vi "Aktuell.vi"() -> ()   [LabVIEW 2012]
uses:
  <vilib>/NXT/Subs/MotorOutput.ctl
  <vilib>/NXT/NXT Controls/ConnectionType.ctl
  <vilib>/NXT/Block Support/NXT_InputPort.ctl
panel:
  out "?":bool
  out "?":bool
  out "?":bool
  out "?":bool
  out "?":bool
  out "Progress":u8(slide) scale=0.0..100.0
  out "Numeric 4":dbl
  out "Numeric 3":dbl
  out "Numeric 2":dbl
  out "Numeric":dbl
  in  "?":bool
  out "?":bool
  out "?":bool
  out "?":bool
  in  "MolekŸlnamen eingeben:":string
  out "Status:":string
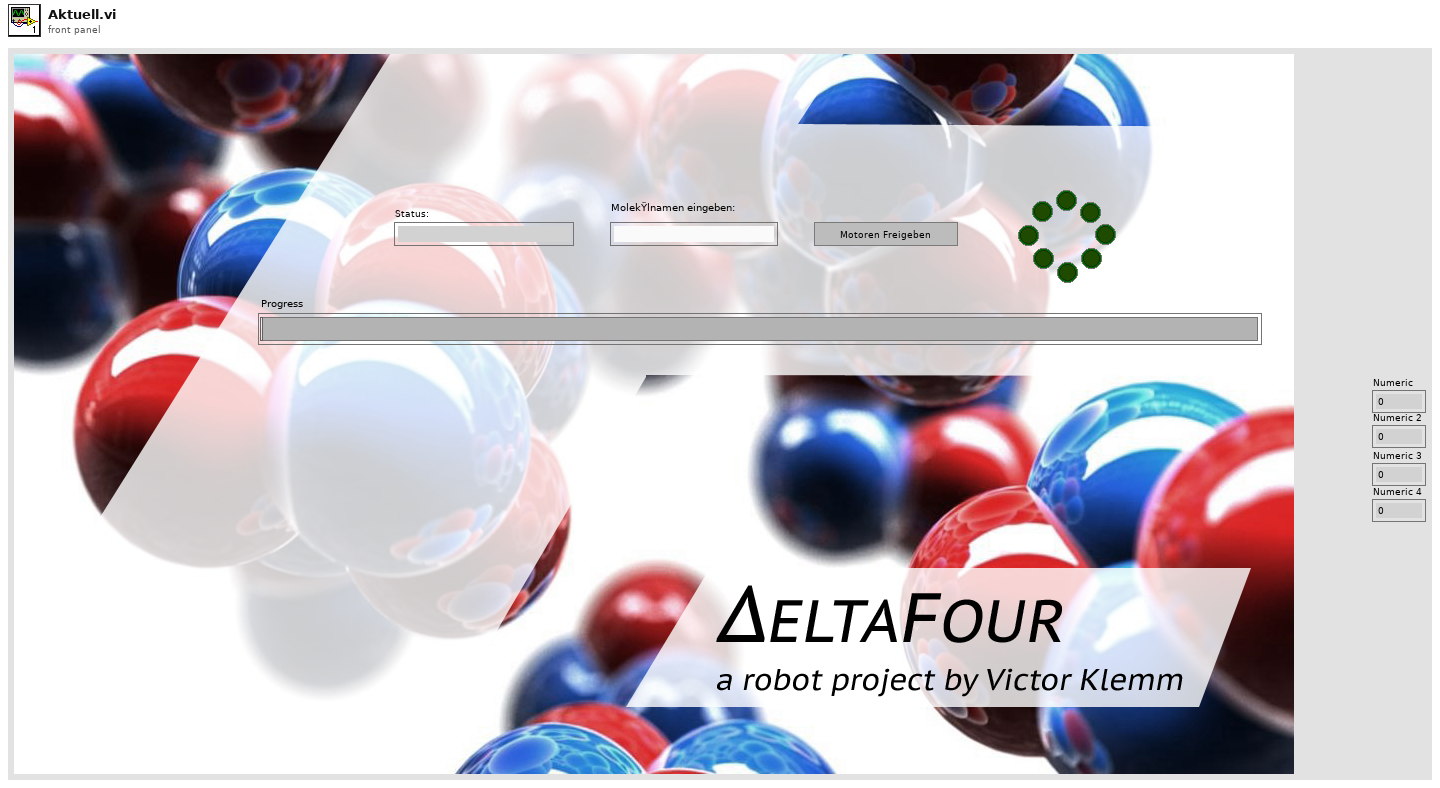
[diagram p1: front panel]
types:
  T1 = typedef "ConnectionType.ctl" = enum16{"Bluetooth", "USB", "WiFi"}
  T2 = typedef "LVHSConnector.ctl" = refnum<class "BrickReference.lvclass">
  T3 = typedef "MotorOutput.ctl" = u8
  T4 = typedef "NXT_InputPort.ctl" = u8
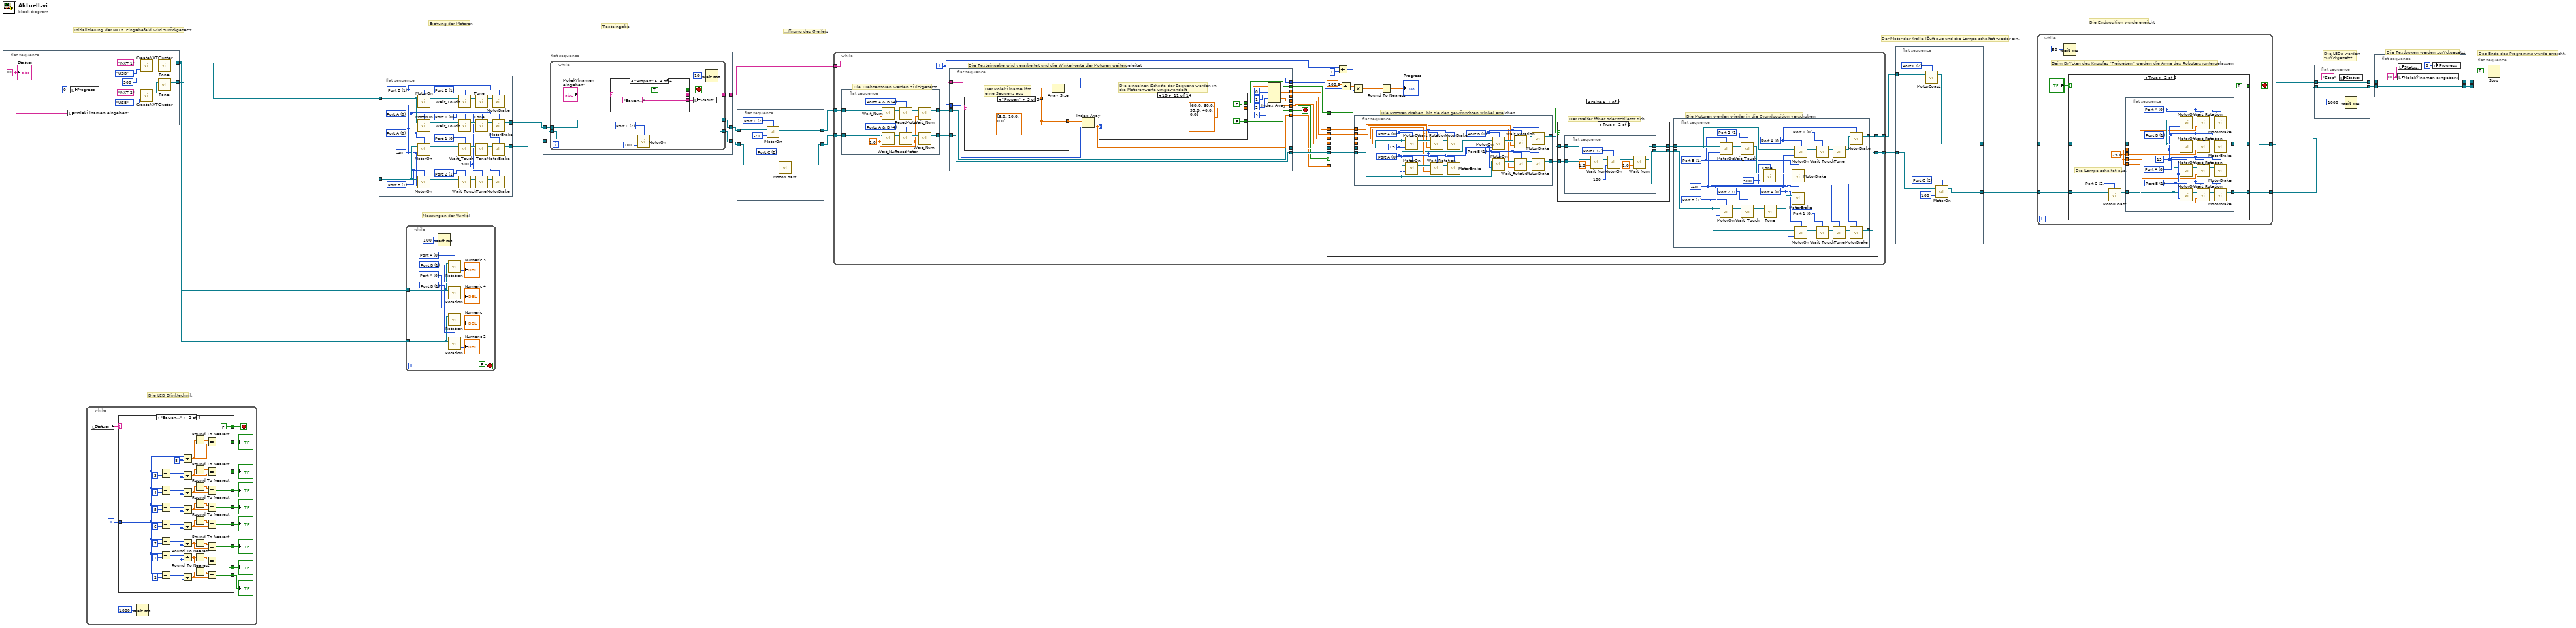
[diagram p0: block diagram]
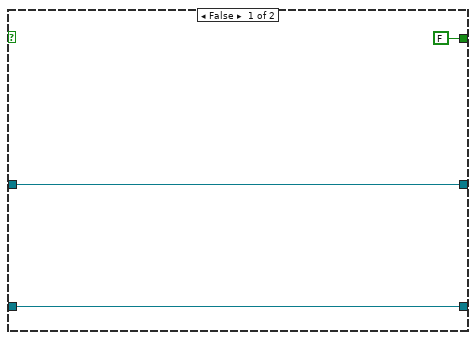
[diagram p2: hidden frame]
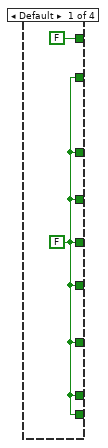
[diagram p3: hidden frame]
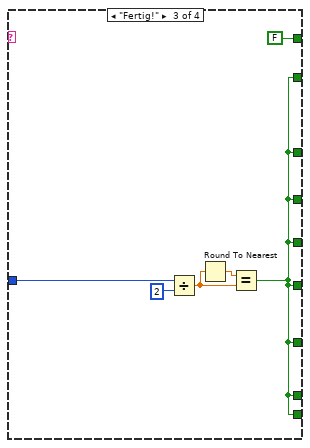
[diagram p4: hidden frame]
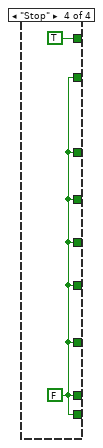
[diagram p5: hidden frame]
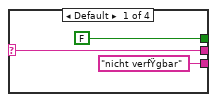
[diagram p6: hidden frame]
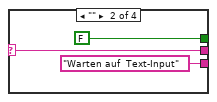
[diagram p7: hidden frame]
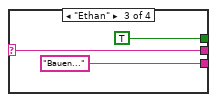
[diagram p8: hidden frame]
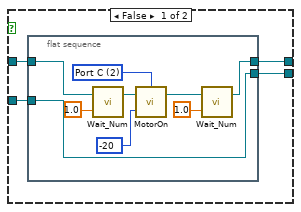
[diagram p9: hidden frame]
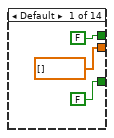
[diagram p11: hidden frame]
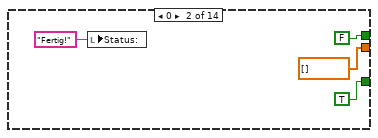
[diagram p12: hidden frame]
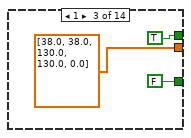
[diagram p13: hidden frame]
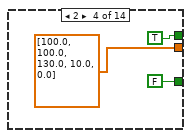
[diagram p14: hidden frame]
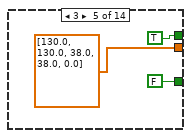
[diagram p15: hidden frame]
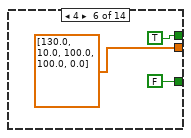
[diagram p16: hidden frame]
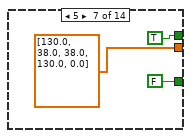
[diagram p17: hidden frame]
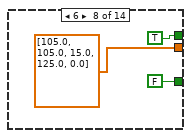
[diagram p18: hidden frame]
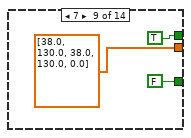
[diagram p19: hidden frame]
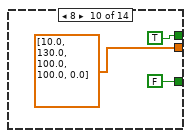
[diagram p20: hidden frame]
diagram:
  # "Der Motor der Kralle lŠuft aus und die Lampe schaltet wieder ein."
  # "Messungen der Winkel"
  # "Die LEDs werden\nzurŸckgesetzt"
  # "Die Textboxen werden zurŸckgesetzt"
  # "Das Ende des Programms wurde erreicht."
  # "Die Endposition wurde erreicht"
  # "…ffnung des Greifers"
  # "Texteingabe"
  # "Eichung der Motoren"
  # "Initialisierung der NXTs. Eingabefeld wird zurŸckgesetzt."
  # "Die LED Blinktechnik"
  n1 = flat-sequence {
    tunnel: [w27] -> w4
    tunnel: [w25] -> w5
    frame #0 {
      w24 = "" ("Status:")
      n2 = local write "MolekŸlnamen eingeben:"(w24) -> ()
      n3 = local write "Progress"(u8 0 ("Progress")) -> ()
      n4 = call <vilib>:"CreateNXTCluster.vi"("Connection Type"=ConnectionType."USB", "NXT name"="NXT 1") -> ("NXT"=w28:T2)  [unwired: 2 in]
      n5 = call <vilib>:"CreateNXTCluster.vi"("Connection Type"=ConnectionType."USB", "NXT name"="NXT 2") -> ("NXT"=w26:T2)  [unwired: 2 in]
      n6 = call <vilib>:"Tone.vi"("NXT"=w28) -> ("NXT"=w27:T2)  [unwired: 3 in]
      n7 = call <vilib>:"Tone.vi"("NXT"=w26, "Tone (440 Hz)"=u16 500) -> ("NXT"=w25:T2)  [unwired: 2 in]
      "Status:" <- w24
    }
  }
  n8 = while {
    i -> [w42]
    stop <- w40 stop-if-true
    n9 = local read "Status:"() -> (w39:string)
    n10 = case shown="\"Bauen...\"" w39 {
      tunnel: w42 -> [_ w46 w88 _]
      tunnel: [FALSE FALSE FALSE TRUE] -> w40
      tunnel: [w43 w74 w86 w92] -> w38
      tunnel: [w43 w73 w86 w92] -> w37
      tunnel: [w43 w72 w86 w92] -> w36
      tunnel: [w43 w67 w86 w92] -> w35
      tunnel: [w43 w63 w86 w92] -> w34
      tunnel: [w43 w57 w86 w92] -> w33
      tunnel: [w43 w52 w86 w92] -> w32
      tunnel: [w43 w47 w86 w92] -> w31
      frame Default {
        w43 = FALSE ("stop? (T)")
      }
      frame "Bauen..." {
        w45 = 8 ("y")
        n11 = Subtract(x=w46, y=3) -> (x-y=w69:i32)
        n12 = Subtract(x=w46, y=4) -> (x-y=w65:i32)
        n13 = Subtract(x=w46, y=5) -> (x-y=w60:i32)
        n14 = Subtract(x=w46, y=6) -> (x-y=w55:i32)
        n15 = Subtract(x=w46, y=7) -> (x-y=w50:i32)
        n16 = Subtract(x=w46, y=1) -> (x-y=w81:i32)
        n17 = Subtract(x=w46, y=2) -> (x-y=w77:i32)
        n18 = Divide(x=w46, y=w45) -> (x/y=w84:dbl)
        n19 = Divide(x=w69, y=w45) -> (x/y=w70:dbl)
        n20 = Divide(x=w65, y=w45) -> (x/y=w66:dbl)
        n21 = Divide(x=w60, y=w45) -> (x/y=w61:dbl)
        n22 = Divide(x=w55, y=w45) -> (x/y=w56:dbl)
        n23 = Divide(x=w50, y=w45) -> (x/y=w51:dbl)
        n24 = Divide(x=w81, y=w45) -> (x/y=w82:dbl)
        n25 = Divide(x=w77, y=w45) -> (x/y=w78:dbl)
        n26 = Round To Nearest(number=w84) -> (nearest integer value=w85:dbl)
        n27 = Round To Nearest(number=w70) -> (nearest integer value=w71:dbl)
        n28 = Round To Nearest(number=w66) -> (nearest integer value=w62:dbl)
        n29 = Round To Nearest(number=w61) -> (nearest integer value=w58:dbl)
        n30 = Round To Nearest(number=w56) -> (nearest integer value=w53:dbl)
        n31 = Round To Nearest(number=w51) -> (nearest integer value=w48:dbl)
        n32 = Round To Nearest(number=w82) -> (nearest integer value=w83:dbl)
        n33 = Round To Nearest(number=w78) -> (nearest integer value=w79:dbl)
        n34 = Equal?(x=w85, y=w84) -> (x = y?=w74:bool)
        n35 = Equal?(x=w71, y=w70) -> (x = y?=w67:bool)
        n36 = Equal?(x=w62, y=w66) -> (x = y?=w63:bool)
        n37 = Equal?(x=w58, y=w61) -> (x = y?=w57:bool)
        n38 = Equal?(x=w53, y=w56) -> (x = y?=w52:bool)
        n39 = Equal?(x=w48, y=w51) -> (x = y?=w47:bool)
        n40 = Equal?(x=w83, y=w82) -> (x = y?=w72:bool)
        n41 = Equal?(x=w79, y=w78) -> (x = y?=w73:bool)
      }
      frame "Fertig!" {
        n42 = Divide(x=w88, y=2) -> (x/y=w90:dbl)
        n43 = Round To Nearest(number=w90) -> (nearest integer value=w87:dbl)
        n44 = Equal?(x=w87, y=w90) -> (x = y?=w86:bool)
      }
      frame "Stop" {
        w92 = FALSE ("stop? (T)")
      }
    }
    "?" <- w38
    "?" <- w37
    "?" <- w36
    "?" <- w32
    "?" <- w31
    "?" <- w35
    "?" <- w34
    "?" <- w33
    n45 = Wait (ms)(milliseconds to wait=u32 1000) -> ()  [unwired: 1 out]
  }
  n46 = flat-sequence {
    tunnel: w5 -> [w115]
    tunnel: w4 -> [w114]
    tunnel: [w101] -> w9
    tunnel: [w100] -> w6
    frame #0 {
      w94 = u16 500 ("Tone (440 Hz)")
      w97 = T3 1 items=["Port A"=0, "Port B"=1, "Port C"=2, "Ports A & B"=4, "Ports A & C"=5, "Ports B & C"=6, "All Ports"=3] ("Output Port (All Ports)")
      w110 = T4 1 items=["Port 1", "Port 2", "Port 3", "Port 4"] ("Port (Port 1)")
      w109 = T4 0 items=["Port 1", "Port 2", "Port 3", "Port 4"] ("Port (Port 1)")
      w95 = T3 1 items=["Port A"=0, "Port B"=1, "Port C"=2, "Ports A & B"=4, "Ports A & C"=5, "Ports B & C"=6, "All Ports"=3] ("Output Port (All Ports)")
      w96 = T3 0 items=["Port A"=0, "Port B"=1, "Port C"=2, "Ports A & B"=4, "Ports A & C"=5, "Ports B & C"=6, "All Ports"=3] ("Output Port (All Ports)")
      w98 = T4 1 items=["Port 1", "Port 2", "Port 3", "Port 4"] ("Port (Port 1)")
      w111 = T4 0 items=["Port 1", "Port 2", "Port 3", "Port 4"] ("Port (Port 1)")
      w102 = -40 ("Power (75)")
      w99 = T3 0 items=["Port A"=0, "Port B"=1, "Port C"=2, "Ports A & B"=4, "Ports A & C"=5, "Ports B & C"=6, "All Ports"=3] ("Output Port (All Ports)")
      n47 = call <vilib>:"MotorOn.vi"("Power (75)"=w102, "NXT"=w114, "Output Port (All Ports)"=w95) -> ("NXT"=w116:T2)  [unwired: 1 in]
      n48 = call <vilib>:"MotorOn.vi"("Power (75)"=w102, "NXT"=w114, "Output Port (All Ports)"=w96) -> ("NXT"=w117:T2)  [unwired: 1 in]
      n49 = call <vilib>:"MotorOn.vi"("Power (75)"=w102, "NXT"=w115, "Output Port (All Ports)"=w99) -> ("NXT"=w119:T2)  [unwired: 1 in]
      n50 = call <vilib>:"MotorOn.vi"("Power (75)"=w102, "NXT"=w115, "Output Port (All Ports)"=w97) -> ("NXT"=w118:T2)  [unwired: 1 in]
      n51 = call <vilib>:"Wait_Touch.vi"("NXT"=w116, "Port (Port 1)"=w110) -> ("NXT"=w106:T2)  [unwired: 2 in]
      n52 = call <vilib>:"Wait_Touch.vi"("NXT"=w117, "Port (Port 1)"=w109) -> ("NXT"=w104:T2)  [unwired: 2 in]
      n53 = call <vilib>:"Wait_Touch.vi"("NXT"=w119, "Port (Port 1)"=w111) -> ("NXT"=w113:T2)  [unwired: 2 in]
      n54 = call <vilib>:"Wait_Touch.vi"("NXT"=w118, "Port (Port 1)"=w98) -> ("NXT"=w108:T2)  [unwired: 2 in]
      n55 = call <vilib>:"Tone.vi"("NXT"=w106) -> ("NXT"=w105:T2)  [unwired: 3 in]
      n56 = call <vilib>:"Tone.vi"("NXT"=w104, "Tone (440 Hz)"=w94) -> ("NXT"=w103:T2)  [unwired: 2 in]
      n57 = call <vilib>:"Tone.vi"("NXT"=w113) -> ("NXT"=w112:T2)  [unwired: 3 in]
      n58 = call <vilib>:"Tone.vi"("NXT"=w108, "Tone (440 Hz)"=w94) -> ("NXT"=w107:T2)  [unwired: 2 in]
      n59 = call <vilib>:"MotorBrake.vi"("NXT"=w105, "Port (All Ports)"=w95) -> ()  [unwired: 2 in, 1 out]
      n60 = call <vilib>:"MotorBrake.vi"("NXT"=w103, "Port (All Ports)"=w96) -> ("NXT"=w100:T2)  [unwired: 2 in]
      n61 = call <vilib>:"MotorBrake.vi"("NXT"=w112, "Port (All Ports)"=w99) -> ("NXT"=w101:T2)  [unwired: 2 in]
      n62 = call <vilib>:"MotorBrake.vi"("NXT"=w107, "Port (All Ports)"=w97) -> ()  [unwired: 2 in, 1 out]
    }
  }
  n63 = while {
    tunnel: w5 -> [w127]
    tunnel: w4 -> [w126]
    stop <- FALSE stop-if-true
    w129 = T3 1 items=["Port A"=0, "Port B"=1, "Port C"=2, "Ports A & B"=4, "Ports A & C"=5, "Ports B & C"=6, "All Ports"=3] ("Output Port (All Ports)")
    w128 = T3 0 items=["Port A"=0, "Port B"=1, "Port C"=2, "Ports A & B"=4, "Ports A & C"=5, "Ports B & C"=6, "All Ports"=3] ("Output Port (All Ports)")
    w131 = T3 1 items=["Port A"=0, "Port B"=1, "Port C"=2, "Ports A & B"=4, "Ports A & C"=5, "Ports B & C"=6, "All Ports"=3] ("Output Port (All Ports)")
    w130 = T3 0 items=["Port A"=0, "Port B"=1, "Port C"=2, "Ports A & B"=4, "Ports A & C"=5, "Ports B & C"=6, "All Ports"=3] ("Output Port (All Ports)")
    n64 = Wait (ms)(milliseconds to wait=u32 100) -> ()  [unwired: 1 out]
    n65 = call <vilib>:"Rotation.vi"("NXT"=w127, "Port (Port A)"=w130) -> ("Angle of Rotation"=→"Numeric 3":i32)  [unwired: 1 in, 1 out]
    n66 = call <vilib>:"Rotation.vi"("NXT"=w127, "Port (Port A)"=w131) -> ("Angle of Rotation"=→"Numeric 4":i32)  [unwired: 1 in, 1 out]
    n67 = call <vilib>:"Rotation.vi"("NXT"=w126, "Port (Port A)"=w128) -> ("Angle of Rotation"=→"Numeric":i32)  [unwired: 1 in, 1 out]
    n68 = call <vilib>:"Rotation.vi"("NXT"=w126, "Port (Port A)"=w129) -> ("Angle of Rotation"=→"Numeric 2":i32)  [unwired: 1 in, 1 out]
  }
  n69 = flat-sequence {
    tunnel: w6 -> [w134]
    tunnel: [w136] -> w19
    tunnel: [w135] -> w18
    tunnel: [w132] -> w17
    tunnel: w9 -> [w133]
    frame #0 {
      n70 = while {
        tunnel: [w144] -> w136
        tunnel: [w141] -> w135
        tunnel: w134 -> [w141]
        tunnel: w133 -> [w138]
        tunnel: [w137] -> w132
        stop <- w142 stop-if-true
        w140 = T3 2 items=["Port A"=0, "Port B"=1, "Port C"=2, "Ports A & B"=4, "Ports A & C"=5, "Ports B & C"=6, "All Ports"=3] ("Output Port (All Ports)")
        n71 = case shown="\"Propan\"" "MolekŸlnamen eingeben:" {
          selector: "MolekŸlnamen eingeben:" -> [w148 w152 w155 w158]
          tunnel: [FALSE FALSE TRUE TRUE] -> w142
          tunnel: [w148 w152 w155 w158] -> w144
          tunnel: ["nicht verfŸgbar" ("Status") "Warten auf  Text-Input" ("Status") "Bauen..." ("Status") "Bauen..." ("Status")] -> w143
          frame Default {
          }
          frame "" {
          }
          frame "Ethan" {
          }
          frame "Propan" {
          }
        }
        n72 = call <vilib>:"MotorOn.vi"("Power (75)"=100, "NXT"=w138, "Output Port (All Ports)"=w140) -> ("NXT"=w137:T2)  [unwired: 1 in]
        n73 = local write "Status:"(w143) -> ()
        n74 = Wait (ms)(milliseconds to wait=u32 10) -> ()  [unwired: 1 out]
      }
    }
  }
  n75 = flat-sequence {
    tunnel: w18 -> [w162]
    tunnel: [w163] -> w8
    tunnel: [w160] -> w7
    tunnel: w17 -> [w161]
    frame #0 {
      w159 = T3 2 items=["Port A"=0, "Port B"=1, "Port C"=2, "Ports A & B"=4, "Ports A & C"=5, "Ports B & C"=6, "All Ports"=3] ("Port (All Ports)")
      w164 = T3 2 items=["Port A"=0, "Port B"=1, "Port C"=2, "Ports A & B"=4, "Ports A & C"=5, "Ports B & C"=6, "All Ports"=3] ("Output Port (All Ports)")
      n76 = call <vilib>:"MotorOn.vi"("Power (75)"=-20, "NXT"=w162, "Output Port (All Ports)"=w164) -> ("NXT"=w163:T2)  [unwired: 1 in]
      n77 = call <vilib>:"MotorCoast.vi"("NXT"=w161, "Port (All Ports)"=w159) -> ("NXT"=w160:T2)  [unwired: 2 in]
    }
  }
  n78 = while {
    tunnel: w8 -> [w183]
    tunnel: w7 -> [w182]
    tunnel: w19 -> [w179]
    tunnel: [w175] -> w16
    tunnel: [w176] -> w3
    i -> [w168]
    stop <- w177 stop-if-true
    # "Die Texteingabe wird verarbeitet und die Winkelwerte der Motoren weitergeleitet"
    # "Die Drehsensoren werden zŸrickgesetzt"
    n79 = flat-sequence {
      tunnel: w183 -> [w350]
      tunnel: [w345] -> w181
      tunnel: [w344] -> w180
      tunnel: w182 -> [w343]
      frame #0 {
        w346 = sgl 1.0 ("Time (1 sec)")
        w352 = T3 4 items=["Port A"=0, "Port B"=1, "Port C"=2, "Ports A & B"=4, "Ports A & C"=5, "Ports B & C"=6, "All Ports"=3] ("Port (All Ports)")
        w353 = T3 4 items=["Port A"=0, "Port B"=1, "Port C"=2, "Ports A & B"=4, "Ports A & C"=5, "Ports B & C"=6, "All Ports"=3] ("Port (All Ports)")
        n80 = call <vilib>:"Wait_Num.vi"("Time (1 sec)"=w346, "NXT"=w350) -> ("NXT"=w349:T2)  [unwired: 2 in]
        n81 = call <vilib>:"Wait_Num.vi"("Time (1 sec)"=w346, "NXT"=w343) -> ("NXT"=w351:T2)  [unwired: 2 in]
        n82 = call <vilib>:"ResetMotor.vi"("NXT"=w349, "Port (All Ports)"=w353) -> ("NXT"=w348:T2)  [unwired: 2 in]
        n83 = call <vilib>:"ResetMotor.vi"("NXT"=w351, "Port (All Ports)"=w352) -> ("NXT"=w347:T2)  [unwired: 2 in]
        n84 = call <vilib>:"Wait_Num.vi"("Time (1 sec)"=w346, "NXT"=w348) -> ("NXT"=w345:T2)  [unwired: 2 in]
        n85 = call <vilib>:"Wait_Num.vi"("Time (1 sec)"=w346, "NXT"=w347) -> ("NXT"=w344:T2)  [unwired: 2 in]
      }
    }
    n86 = flat-sequence {
      tunnel: [w292] -> w189
      tunnel: [w291] -> w188
      tunnel: [w290] -> w187
      tunnel: [w289] -> w186
      tunnel: [w284] -> w185
      tunnel: w181 -> [w284]
      tunnel: w180 -> [w288]
      tunnel: [w288] -> w184
      tunnel: w179 -> [w287]
      tunnel: w168 -> [w281]
      tunnel: [w285] -> w177
      tunnel: [w282] -> w178
      tunnel: [w280] -> w174
      tunnel: [w278] -> w169
      frame #0 {
        # "Die einzelnen Schritte der Sequenz werden in\ndie Motorenwerte umgewandelt"
        # "Der MolekŸlname lšst eine Sequenz aus"
        n87 = case shown="\"Propan\"" w287 {
          tunnel: [w340 w341 w342] -> w286
          tunnel: [w340 w341 w342] -> w279
          frame Default {
            w340 = dbl[] [0.0] ("array")
          }
          frame "Ethan" {
            w341 = dbl[] [8.0, 10.0, 2.0, 11.0, 0.0] ("array")
          }
          frame "Propan" {
            w342 = dbl[] [6.0, 10.0, 0.0] ("array")
          }
        }
        n88 = Array Size(array=w279) -> (size(s)=w278:i32)
        n89 = Index Array(array=w286, index=w281) -> (element=w280:dbl)
        n90 = case shown="10" w280 {
          tunnel: [FALSE TRUE FALSE FALSE FALSE FALSE FALSE FALSE FALSE FALSE FALSE FALSE FALSE FALSE] -> w285
          tunnel: [dbl[] [] ("array") dbl[] [] ("array") dbl[] [38.0, 38.0, 130.0, 130.0, 0.0] ("array") dbl[] [100.0, 100.0, 130.0, 10.0, 0.0] ("array") dbl[] [130.0, 130.0, 38.0, 38.0, 0.0] ("array") dbl[] [130.0, 10.0, 100.0, 100.0, 0.0] ("array") dbl[] [130.0, 38.0, 38.0, 130.0, 0.0] ("array") dbl[] [105.0, 105.0, 15.0, 125.0, 0.0] ("array") dbl[] [38.0, 130.0, 38.0, 130.0, 0.0] ("array") dbl[] [10.0, 130.0, 100.0, 100.0, 0.0] ("array") dbl[] [60.0, 60.0, 35.0, 40.0, 0.0] ("array") dbl[] [0.0, 0.0, 0.0, 0.0, 0.0] ("array") dbl[] [0.0, 0.0, 0.0, 0.0, 0.0] ("array") dbl[] [0.0, 0.0, 0.0, 0.0, 0.0] ("array")] -> w283
          tunnel: [FALSE FALSE TRUE TRUE TRUE TRUE TRUE TRUE TRUE TRUE FALSE FALSE FALSE FALSE] -> w282
          frame Default {
          }
          frame 0 {
            n91 = local write "Status:"("Fertig!" ("Status:")) -> ()
          }
          frame 1 {
          }
          frame 2 {
          }
          frame 3 {
          }
          frame 4 {
          }
          frame 5 {
          }
          frame 6 {
          }
          frame 7 {
          }
          frame 8 {
          }
          frame 10 {
          }
          frame 11 {
          }
          frame 12 {
          }
          frame 13 {
          }
        }
        n92 = Index Array(array=w283, index #1=0 ("index"), index #2=1 ("index"), index #3=2 ("index"), index #4=3 ("index")) -> (element #1=w291:dbl, element #2=w290:dbl, element #3=w289:dbl, element #4=w292:dbl)
      }
    }
    n93 = case shown="False" w177 {
      tunnel: w189 -> [w196 _]
      tunnel: w188 -> [w199 _]
      tunnel: w187 -> [w198 _]
      tunnel: w186 -> [w197 _]
      tunnel: w185 -> [w195 w277]
      tunnel: w184 -> [w194 w276]
      tunnel: [w193 w277] -> w175
      tunnel: [w192 w276] -> w176
      tunnel: w178 -> [w200 _]
      tunnel: w174 -> [_ _]
      frame False {
        # "Die Motoren drehen, bis sie den gewŸnschten Winkel erreichen"
        # "Der Greifer šffnet oder schliesst sich"
        # "Die Motoren werden wieder in die Grundposition verschoben"
        n94 = flat-sequence {
          tunnel: w194 -> [w249]
          tunnel: w195 -> [w229]
          tunnel: [w236] -> w201
          tunnel: [w235] -> w202
          tunnel: w199 -> [w233]
          tunnel: w198 -> [w232]
          tunnel: w197 -> [w231]
          tunnel: w196 -> [w230]
          frame #0 {
            w234 = 15 ("Power (75)")
            w240 = T3 1 items=["Port A"=0, "Port B"=1, "Port C"=2, "Ports A & B"=4, "Ports A & C"=5, "Ports B & C"=6, "All Ports"=3] ("Output Port (All Ports)")
            w239 = T3 0 items=["Port A"=0, "Port B"=1, "Port C"=2, "Ports A & B"=4, "Ports A & C"=5, "Ports B & C"=6, "All Ports"=3] ("Output Port (All Ports)")
            w237 = T3 1 items=["Port A"=0, "Port B"=1, "Port C"=2, "Ports A & B"=4, "Ports A & C"=5, "Ports B & C"=6, "All Ports"=3] ("Output Port (All Ports)")
            w241 = T3 0 items=["Port A"=0, "Port B"=1, "Port C"=2, "Ports A & B"=4, "Ports A & C"=5, "Ports B & C"=6, "All Ports"=3] ("Output Port (All Ports)")
            n95 = call <vilib>:"MotorOn.vi"("Power (75)"=w234, "NXT"=w229, "Output Port (All Ports)"=w239) -> ("NXT"=w246:T2)  [unwired: 1 in]
            n96 = call <vilib>:"MotorOn.vi"("Power (75)"=w234, "NXT"=w249, "Output Port (All Ports)"=w241) -> ("NXT"=w248:T2)  [unwired: 1 in]
            n97 = call <vilib>:"Wait_Rotation.vi"("Position Change (180)"=w233, "NXT"=w246, "Port (Port A)"=w239) -> ("NXT"=w244:T2)  [unwired: 1 in]
            n98 = call <vilib>:"Wait_Rotation.vi"("Position Change (180)"=w231, "NXT"=w248, "Port (Port A)"=w241) -> ("NXT"=w242:T2)  [unwired: 1 in]
            n99 = call <vilib>:"MotorBrake.vi"("NXT"=w244, "Port (All Ports)"=w239) -> ()  [unwired: 2 in, 1 out]
            n100 = call <vilib>:"MotorBrake.vi"("NXT"=w242, "Port (All Ports)"=w241) -> ()  [unwired: 2 in, 1 out]
            n101 = call <vilib>:"MotorOn.vi"("Power (75)"=w234, "NXT"=w229, "Output Port (All Ports)"=w240) -> ("NXT"=w247:T2)  [unwired: 1 in]
            n102 = call <vilib>:"MotorOn.vi"("Power (75)"=w234, "NXT"=w249, "Output Port (All Ports)"=w237) -> ("NXT"=w245:T2)  [unwired: 1 in]
            n103 = call <vilib>:"Wait_Rotation.vi"("Position Change (180)"=w232, "NXT"=w247, "Port (Port A)"=w240) -> ("NXT"=w243:T2)  [unwired: 1 in]
            n104 = call <vilib>:"Wait_Rotation.vi"("Position Change (180)"=w230, "NXT"=w245, "Port (Port A)"=w237) -> ("NXT"=w238:T2)  [unwired: 1 in]
            n105 = call <vilib>:"MotorBrake.vi"("NXT"=w243, "Port (All Ports)"=w240) -> ("NXT"=w235:T2)  [unwired: 2 in]
            n106 = call <vilib>:"MotorBrake.vi"("NXT"=w238, "Port (All Ports)"=w237) -> ("NXT"=w236:T2)  [unwired: 2 in]
          }
        }
        n107 = case shown="True" w200 {
          tunnel: w202 -> [w206 w219]
          tunnel: w201 -> [w205 w218]
          tunnel: [w204 w217] -> w191
          tunnel: [w203 w216] -> w190
          frame False {
            n108 = flat-sequence {
              tunnel: [w207] -> w204
              tunnel: [w210] -> w203
              tunnel: w206 -> [w212]
              tunnel: w205 -> [w210]
              frame #0 {
                w214 = T3 2 items=["Port A"=0, "Port B"=1, "Port C"=2, "Ports A & B"=4, "Ports A & C"=5, "Ports B & C"=6, "All Ports"=3] ("Output Port (All Ports)")
                n109 = call <vilib>:"Wait_Num.vi"("Time (1 sec)"=sgl 1.0, "NXT"=w212) -> ("NXT"=w211:T2)  [unwired: 2 in]
                n110 = call <vilib>:"MotorOn.vi"("Power (75)"=-20, "NXT"=w211, "Output Port (All Ports)"=w214) -> ("NXT"=w208:T2)  [unwired: 1 in]
                n111 = call <vilib>:"Wait_Num.vi"("Time (1 sec)"=sgl 1.0, "NXT"=w208) -> ("NXT"=w207:T2)  [unwired: 2 in]
              }
            }
          }
          frame True {
            n112 = flat-sequence {
              tunnel: w218 -> [w222]
              tunnel: [w221] -> w217
              tunnel: w219 -> [w225]
              tunnel: [w222] -> w216
              frame #0 {
                w226 = T3 2 items=["Port A"=0, "Port B"=1, "Port C"=2, "Ports A & B"=4, "Ports A & C"=5, "Ports B & C"=6, "All Ports"=3] ("Output Port (All Ports)")
                n113 = call <vilib>:"Wait_Num.vi"("Time (1 sec)"=sgl 1.0, "NXT"=w225) -> ("NXT"=w224:T2)  [unwired: 2 in]
                n114 = call <vilib>:"MotorOn.vi"("Power (75)"=100, "NXT"=w224, "Output Port (All Ports)"=w226) -> ("NXT"=w220:T2)  [unwired: 1 in]
                n115 = call <vilib>:"Wait_Num.vi"("Time (1 sec)"=sgl 1.0, "NXT"=w220) -> ("NXT"=w221:T2)  [unwired: 2 in]
              }
            }
          }
        }
        n116 = flat-sequence {
          tunnel: w191 -> [w271]
          tunnel: w190 -> [w270]
          tunnel: [w257] -> w193
          tunnel: [w256] -> w192
          frame #0 {
            w250 = u16 500 ("Tone (440 Hz)")
            w253 = T3 1 items=["Port A"=0, "Port B"=1, "Port C"=2, "Ports A & B"=4, "Ports A & C"=5, "Ports B & C"=6, "All Ports"=3] ("Output Port (All Ports)")
            w266 = T4 1 items=["Port 1", "Port 2", "Port 3", "Port 4"] ("Port (Port 1)")
            w265 = T4 0 items=["Port 1", "Port 2", "Port 3", "Port 4"] ("Port (Port 1)")
            w251 = T3 1 items=["Port A"=0, "Port B"=1, "Port C"=2, "Ports A & B"=4, "Ports A & C"=5, "Ports B & C"=6, "All Ports"=3] ("Output Port (All Ports)")
            w252 = T3 0 items=["Port A"=0, "Port B"=1, "Port C"=2, "Ports A & B"=4, "Ports A & C"=5, "Ports B & C"=6, "All Ports"=3] ("Output Port (All Ports)")
            w254 = T4 1 items=["Port 1", "Port 2", "Port 3", "Port 4"] ("Port (Port 1)")
            w267 = T4 0 items=["Port 1", "Port 2", "Port 3", "Port 4"] ("Port (Port 1)")
            w258 = -40 ("Power (75)")
            w255 = T3 0 items=["Port A"=0, "Port B"=1, "Port C"=2, "Ports A & B"=4, "Ports A & C"=5, "Ports B & C"=6, "All Ports"=3] ("Output Port (All Ports)")
            n117 = call <vilib>:"MotorOn.vi"("Power (75)"=w258, "NXT"=w271, "Output Port (All Ports)"=w253) -> ("NXT"=w274:T2)  [unwired: 1 in]
            n118 = call <vilib>:"MotorOn.vi"("Power (75)"=w258, "NXT"=w270, "Output Port (All Ports)"=w251) -> ("NXT"=w272:T2)  [unwired: 1 in]
            n119 = call <vilib>:"Wait_Touch.vi"("NXT"=w274, "Port (Port 1)"=w254) -> ("NXT"=w264:T2)  [unwired: 2 in]
            n120 = call <vilib>:"Wait_Touch.vi"("NXT"=w272, "Port (Port 1)"=w266) -> ("NXT"=w262:T2)  [unwired: 2 in]
            n121 = call <vilib>:"Tone.vi"("NXT"=w264, "Tone (440 Hz)"=w250) -> ("NXT"=w263:T2)  [unwired: 2 in]
            n122 = call <vilib>:"Tone.vi"("NXT"=w262) -> ("NXT"=w261:T2)  [unwired: 3 in]
            n123 = call <vilib>:"MotorBrake.vi"("NXT"=w263, "Port (All Ports)"=w253) -> ()  [unwired: 2 in, 1 out]
            n124 = call <vilib>:"MotorBrake.vi"("NXT"=w261, "Port (All Ports)"=w251) -> ()  [unwired: 2 in, 1 out]
            n125 = call <vilib>:"MotorOn.vi"("Power (75)"=w258, "NXT"=w271, "Output Port (All Ports)"=w255) -> ("NXT"=w275:T2)  [unwired: 1 in]
            n126 = call <vilib>:"MotorOn.vi"("Power (75)"=w258, "NXT"=w270, "Output Port (All Ports)"=w252) -> ("NXT"=w273:T2)  [unwired: 1 in]
            n127 = call <vilib>:"Wait_Touch.vi"("NXT"=w275, "Port (Port 1)"=w267) -> ("NXT"=w269:T2)  [unwired: 2 in]
            n128 = call <vilib>:"Wait_Touch.vi"("NXT"=w273, "Port (Port 1)"=w265) -> ("NXT"=w260:T2)  [unwired: 2 in]
            n129 = call <vilib>:"Tone.vi"("NXT"=w269) -> ("NXT"=w268:T2)  [unwired: 3 in]
            n130 = call <vilib>:"Tone.vi"("NXT"=w260, "Tone (440 Hz)"=w250) -> ("NXT"=w259:T2)  [unwired: 2 in]
            n131 = call <vilib>:"MotorBrake.vi"("NXT"=w268, "Port (All Ports)"=w255) -> ("NXT"=w257:T2)  [unwired: 2 in]
            n132 = call <vilib>:"MotorBrake.vi"("NXT"=w259, "Port (All Ports)"=w252) -> ("NXT"=w256:T2)  [unwired: 2 in]
          }
        }
      }
      frame True {
      }
    }
    n133 = Add(x=w168, y=1) -> (x+y=w166:i32)
    n134 = Divide(x=100.0 ("y"), y=w169) -> (x/y=w172:dbl)
    n135 = Multiply(x=w172, y=w166) -> (x*y=w171:dbl)
    n136 = Round To Nearest(number=w171) -> (nearest integer value=→"Progress":dbl)
  }
  n137 = flat-sequence {
    tunnel: w16 -> [w360]
    tunnel: [w358] -> w15
    tunnel: w3 -> [w355]
    tunnel: [w354] -> w2
    frame #0 {
      w356 = T3 2 items=["Port A"=0, "Port B"=1, "Port C"=2, "Ports A & B"=4, "Ports A & C"=5, "Ports B & C"=6, "All Ports"=3] ("Output Port (All Ports)")
      w359 = T3 2 items=["Port A"=0, "Port B"=1, "Port C"=2, "Ports A & B"=4, "Ports A & C"=5, "Ports B & C"=6, "All Ports"=3] ("Output Port (All Ports)")
      n138 = call <vilib>:"MotorCoast.vi"("NXT"=w360, "Port (All Ports)"=w359) -> ("NXT"=w358:T2)  [unwired: 2 in]
      n139 = call <vilib>:"MotorOn.vi"("Power (75)"=100, "NXT"=w355, "Output Port (All Ports)"=w356) -> ("NXT"=w354:T2)  [unwired: 1 in]
    }
  }
  n140 = while {
    tunnel: w15 -> [w364]
    tunnel: w2 -> [w363]
    tunnel: [w362] -> w1
    tunnel: [w361] -> w14
    stop <- w365 stop-if-true
    # "Beim DrŸcken des Knopfes \"Freigeben\" werden die Arme des Roboters runtergelassen"
    n141 = Wait (ms)(milliseconds to wait=u32 50) -> ()  [unwired: 1 out]
    n142 = case shown="True" "?" {
      tunnel: w364 -> [w369 w378]
      tunnel: w363 -> [w368 w372]
      tunnel: [FALSE TRUE] -> w365
      tunnel: [w369 w375] -> w362
      tunnel: [w368 w374] -> w361
      frame False {
      }
      frame True {
        w373 = T3 2 items=["Port A"=0, "Port B"=1, "Port C"=2, "Ports A & B"=4, "Ports A & C"=5, "Ports B & C"=6, "All Ports"=3] ("Port (All Ports)")
        w377 = 25.0
        # "Die Lampe schaltet aus."
        n143 = call <vilib>:"MotorCoast.vi"("NXT"=w372, "Port (All Ports)"=w373) -> ("NXT"=w371:T2)  [unwired: 2 in]
        n144 = flat-sequence {
          tunnel: w378 -> [w399]
          tunnel: [w386] -> w375
          tunnel: [w385] -> w374
          tunnel: w377 -> [w383]
          tunnel: w377 -> [w382]
          tunnel: w377 -> [w381]
          tunnel: w377 -> [w380]
          tunnel: w371 -> [w379]
          frame #0 {
            w384 = 15 ("Power (75)")
            w390 = T3 1 items=["Port A"=0, "Port B"=1, "Port C"=2, "Ports A & B"=4, "Ports A & C"=5, "Ports B & C"=6, "All Ports"=3] ("Output Port (All Ports)")
            w389 = T3 0 items=["Port A"=0, "Port B"=1, "Port C"=2, "Ports A & B"=4, "Ports A & C"=5, "Ports B & C"=6, "All Ports"=3] ("Output Port (All Ports)")
            w387 = T3 1 items=["Port A"=0, "Port B"=1, "Port C"=2, "Ports A & B"=4, "Ports A & C"=5, "Ports B & C"=6, "All Ports"=3] ("Output Port (All Ports)")
            w391 = T3 0 items=["Port A"=0, "Port B"=1, "Port C"=2, "Ports A & B"=4, "Ports A & C"=5, "Ports B & C"=6, "All Ports"=3] ("Output Port (All Ports)")
            n145 = call <vilib>:"MotorOn.vi"("Power (75)"=w384, "NXT"=w399, "Output Port (All Ports)"=w391) -> ("NXT"=w398:T2)  [unwired: 1 in]
            n146 = call <vilib>:"MotorOn.vi"("Power (75)"=w384, "NXT"=w399, "Output Port (All Ports)"=w387) -> ("NXT"=w395:T2)  [unwired: 1 in]
            n147 = call <vilib>:"MotorOn.vi"("Power (75)"=w384, "NXT"=w379, "Output Port (All Ports)"=w389) -> ("NXT"=w396:T2)  [unwired: 1 in]
            n148 = call <vilib>:"MotorOn.vi"("Power (75)"=w384, "NXT"=w379, "Output Port (All Ports)"=w390) -> ("NXT"=w397:T2)  [unwired: 1 in]
            n149 = call <vilib>:"Wait_Rotation.vi"("Position Change (180)"=w381, "NXT"=w398, "Port (Port A)"=w391) -> ("NXT"=w392:T2)  [unwired: 1 in]
            n150 = call <vilib>:"Wait_Rotation.vi"("Position Change (180)"=w380, "NXT"=w395, "Port (Port A)"=w387) -> ("NXT"=w388:T2)  [unwired: 1 in]
            n151 = call <vilib>:"Wait_Rotation.vi"("Position Change (180)"=w383, "NXT"=w396, "Port (Port A)"=w389) -> ("NXT"=w394:T2)  [unwired: 1 in]
            n152 = call <vilib>:"Wait_Rotation.vi"("Position Change (180)"=w382, "NXT"=w397, "Port (Port A)"=w390) -> ("NXT"=w393:T2)  [unwired: 1 in]
            n153 = call <vilib>:"MotorBrake.vi"("NXT"=w392, "Port (All Ports)"=w391) -> ()  [unwired: 2 in, 1 out]
            n154 = call <vilib>:"MotorBrake.vi"("NXT"=w388, "Port (All Ports)"=w387) -> ("NXT"=w386:T2)  [unwired: 2 in]
            n155 = call <vilib>:"MotorBrake.vi"("NXT"=w394, "Port (All Ports)"=w389) -> ()  [unwired: 2 in, 1 out]
            n156 = call <vilib>:"MotorBrake.vi"("NXT"=w393, "Port (All Ports)"=w390) -> ("NXT"=w385:T2)  [unwired: 2 in]
          }
        }
      }
    }
  }
  n157 = flat-sequence {
    tunnel: [w402] -> w10
    tunnel: w1 -> [w402]
    tunnel: [w401] -> w12
    tunnel: w14 -> [w401]
    frame #0 {
      n158 = local write "Status:"("Stop" ("Status:")) -> ()
      n159 = Wait (ms)(milliseconds to wait=u32 1000) -> ()  [unwired: 1 out]
    }
  }
  n160 = flat-sequence {
    tunnel: [w407] -> w13
    tunnel: w12 -> [w407]
    tunnel: [w406] -> w11
    tunnel: w10 -> [w406]
    frame #0 {
      w405 = "" ("Status:")
      n161 = local write "MolekŸlnamen eingeben:"(w405) -> ()
      n162 = local write "Status:"(w405) -> ()
      n163 = local write "Progress"(u8 0 ("Progress")) -> ()
    }
  }
  n164 = flat-sequence {
    tunnel: w13 -> [_]
    tunnel: w11 -> [_]
    frame #0 {
      n165 = Stop(stop? (T)=TRUE) -> ()
    }
  }
